vi "stft.vi"(0 "array":waveform(dbl)[](array[waveform])) -> (12 "power spectra [dB EU] 3":dbl[][](array[numeric]) format="%.2f", 13 "power spectra [dB EU] 4":dbl[][](array[numeric]) format="%.2f", 14 "input1":waveform(dbl), 15 "input3":waveform(dbl), 16 "input2":waveform(dbl), 17 "power spectra [dB EU]":dbl[][](array[numeric]) format="%.2f", 18 "input4":waveform(dbl), 19 "power spectra [dB EU] 2":dbl[][](array[numeric]) format="%.2f")   [LabVIEW 2021]
uses:
  <vilib>/addons/Sound and Vibration/svt_Transients/SVT STFT vs Time (Intensity).vi
  <vilib>/addons/Sound and Vibration/svt_Transients/SoundVib_Transient.lvlib
panel:
  out "f0 and delta f [Hz]":cluster{"f0":dbl, "delta f":dbl}={"f0"=0.0, "delta f"=0.0009765625} {"delta f" format="%.2f"; "f0" format="%.2f"}
  out "t0 and delta t [s]":cluster{"t0":dbl, "delta t":dbl} {"delta t" format="%.2f"; "t0" format="%.2f"}
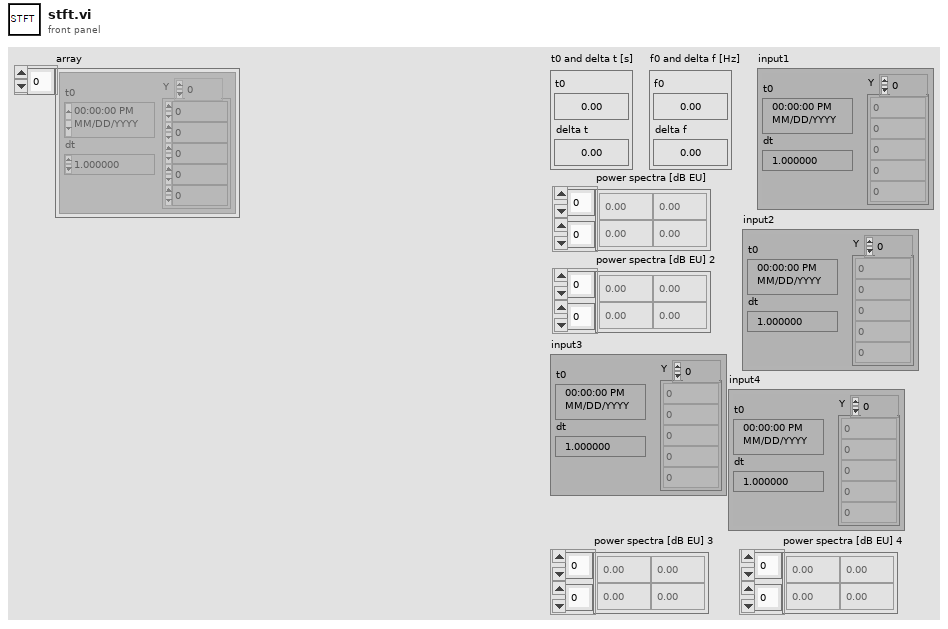
[diagram p1: front panel]
types:
  T1 = cluster{"from [s]":dbl, "to [s]":dbl, "time increment":dbl, "time increment units (%)":enum16{"%", "s", "ms"}}
  T2 = enum16{"None ", "Hanning", "Hamming", "Blackman-Harris", "Exact Blackman", "Blackman", "Flat Top", "4 Term B-Harris ", "7 Term B-Harris", "Low Sidelobe"}
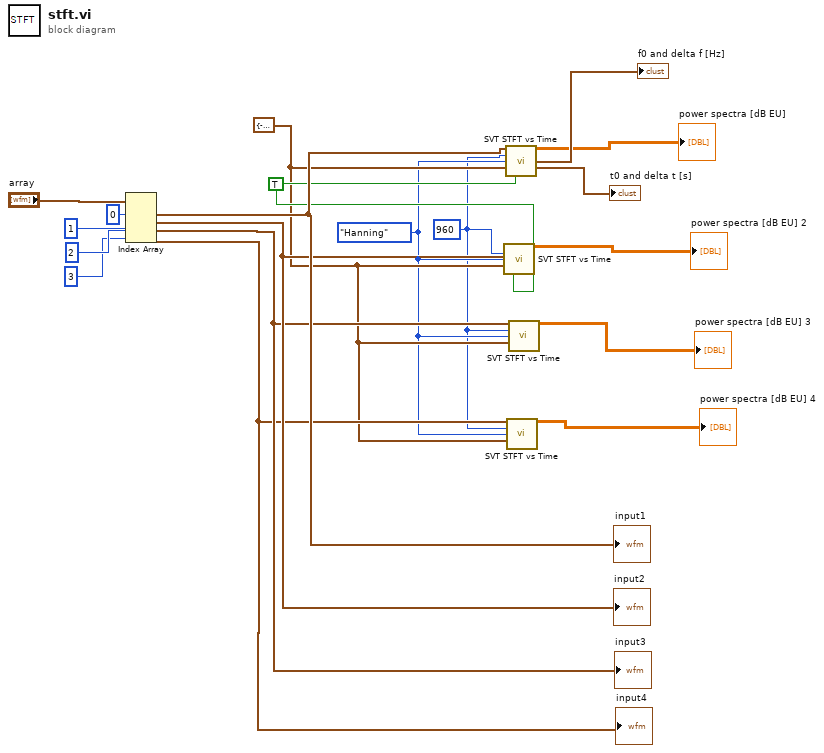
[diagram p0: block diagram]
diagram:
  w5 = T1 {"from [s]"=-1.0, "to [s]"=-1.0, "time increment"=1.0, "time increment units (%)"=enum."%"} ("time segment")
  w15 = TRUE ("dB On (T)")
  w4 = T2."Hanning" ("window")
  w3 = 960 ("FFT block size")
  n1 = Index Array(array="array", index #1=0 ("index"), index #2=1 ("index"), index #3=2 ("index"), index #4=3 ("index")) -> (element #1=w19:waveform(dbl), element #2=w16:waveform(dbl), element #3=w7:waveform(dbl), element #4=w6:waveform(dbl))
  "input1" <- w19
  "input2" <- w16
  "input3" <- w7
  "input4" <- w6
  n2 = call-poly <vilib>:"SVT STFT vs Time.vi"("scaled signal [EU]"=w16, "FFT block size"=w3, "window"=w4, "time segment"=w5, "dB On (T)"=w15) -> ("power spectra [dB EU]"=→"power spectra [dB EU] 2":dbl[][])  [unwired: 5 in, 5 out]
  n3 = call-poly <vilib>:"SVT STFT vs Time.vi"("scaled signal [EU]"=w19, "FFT block size"=w3, "window"=w4, "time segment"=w5, "dB On (T)"=w15) -> ("power spectra [dB EU]"=→"power spectra [dB EU]":dbl[][], "f0 and delta f [Hz]"=→"f0 and delta f [Hz]":cluster{"f0":dbl, "delta f":dbl}, "t0 and delta t [s]"=→"t0 and delta t [s]":cluster{"t0":dbl, "delta t":dbl})  [unwired: 5 in, 3 out]
  n4 = call-poly <vilib>:"SVT STFT vs Time.vi"("scaled signal [EU]"=w6, "FFT block size"=w3, "window"=w4, "time segment"=w5) -> ("power spectra [dB EU]"=→"power spectra [dB EU] 4":dbl[][])  [unwired: 6 in, 5 out]
  n5 = call-poly <vilib>:"SVT STFT vs Time.vi"("scaled signal [EU]"=w7, "FFT block size"=w3, "window"=w4, "time segment"=w5) -> ("power spectra [dB EU]"=→"power spectra [dB EU] 3":dbl[][])  [unwired: 6 in, 5 out]
